vi "BRig_RT__Case_Exp__State_CuePre.vi"(0 "input_dataCurrent":u16[](array[numeric]), 1 "input_dataTrial":u16[][](array[numeric]), 6 "input_I_lick":bool, 7 "input_dataExp":u16[](array[numeric]), 9 "input_arrTrig":bool[](array[boolean])) -> (12 "output_state":T1, 13 "output_arrTrig":bool[](array[boolean]), 14 "output_dataCurrent":u16[](array[numeric]), 15 "output_dataTrial":u16[][](array[numeric]))   [LabVIEW 2014]
uses:
  myRIO_BRig_RT__Case_Exp_stateList.ctl
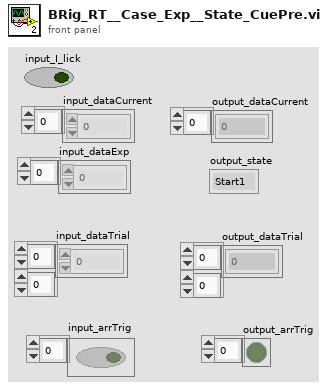
[diagram p1: front panel]
types:
  T1 = typedef "myRIO_BRig_RT__Case_Exp_stateList.ctl" = enum16{"Start1", "Start2", "Start3", "saveSettings1", "saveSettings2", "saveSettings3", "saveSettings4", "saveSettings_LC_ENL_l1", "saveSettings_LC_ENL_l2", "saveSettings_LC_Cue_l1", "saveSettings_LC_Cue_l2", "saveSettings6_LC_l1_Other", "SaveSettings6_LC_l2_Other", "setSettings_Audio", "setSettings_Laser", "initBlock_pre", "initBlock", "initBlock2", "initBlock_post", "initTrial_pre", "initTrial", "initTrial2", "initTrial3", "initTrial4", "initTrial_LC_ENL1", "initTrial_LC_Cue1", "initTrial_LC_Cue1_2", "initTrial_LC_Sel", "initTrial_post", "ENL1_pre", "ENL1", "ENL1_post", "ENL1Penalty_pre", "ENL1Penalty", "ENL2_pre", "ENL2", "ENL2Penalty_pre", "ENL2Penalty", "Cue1_pre", "Cue1", "Cue1_post", "Cue1Penalty_pre", "Cue1Penalty", "Cue2_pre", "Cue2", "Cue2Penalty_pre", "Cue2Penalty", "Selection_pre", "Selection", "Select_post", "SelectReward_pre", "SelectReward", "SelectRewardPost_pre", "SelectRewardPost", "SelectWrong_pre", "SelectWrong", "SelectWrong_post", "SelectTimeout_pre", "SelectTimeout", "SelectTimeout_post", "endTrial_pre", "endTrial1", "endTrial2", "endTrial3", "endTrial_post", "endBlock_pre", "endBlock", "endBlock_post", "endExp", "commConnect", "commUpload_pre", "commUpload_dataBlock", "commUpload_dataCurrent", "commUpload_dataExp", "commUpload_dataLC", "commUpload_dataTrial", "commUpload_post", "saveData_pre", "saveData_dataBlock", "saveData_dataCurrent", "saveData_dataExp", "saveData_dataLC", "saveData_dataTrial", "saveData_post", "empty_endBlock1", "empty_endBlock2", "empty_endTrial1", "empty_endTrial2", "empty_endTrial3", "empty_endTrial4", "empty_endTrial5", "dummyState", "dummyState_endBlock", "FreeReward_pre", "FreeReward", "FreeRewardPost_pre", "FreeRewardPost"}
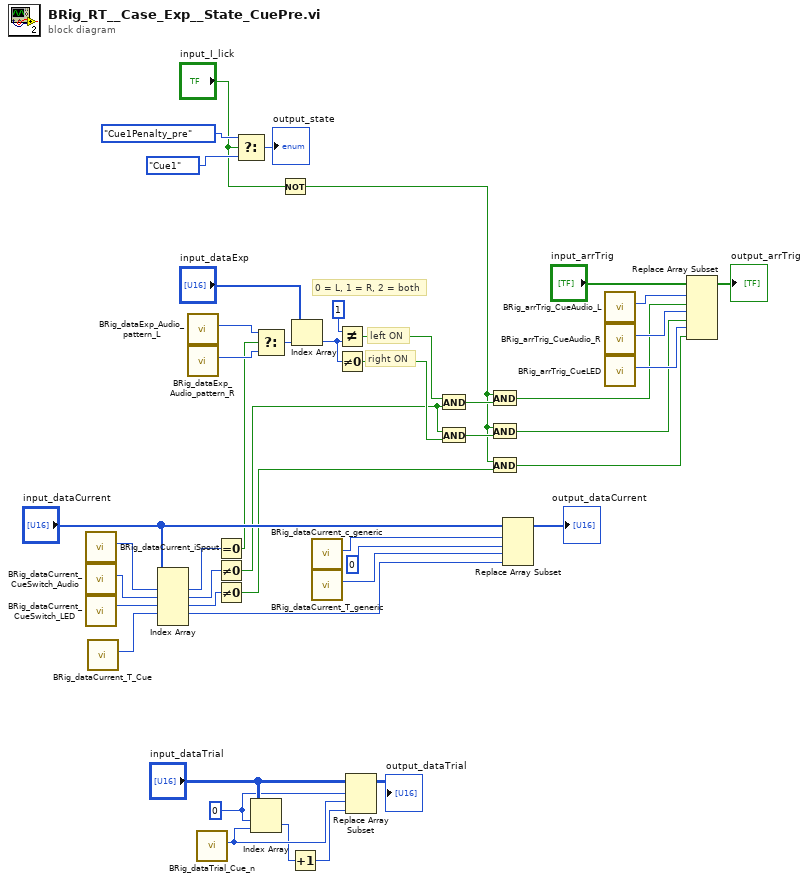
[diagram p0: block diagram]
diagram:
  w1 = 0
  # "right ON"
  # "left ON"
  # "0 = L, 1 = R, 2 = both"
  n1 = call "BRig_dataCurrent_iSpout.vi"() -> ("output_iSpout"=w24:i32)  [unwired: 11 in]
  n2 = call "BRig_dataCurrent_CueSwitch_Audio.vi"() -> ("output_CueSwitch_Audio"=w28:i32)  [unwired: 11 in]
  n3 = call "BRig_dataCurrent_CueSwitch_LED.vi"() -> ("output_CueSwitch_LED"=w29:i32)  [unwired: 11 in]
  n4 = call "BRig_dataCurrent_T_Cue.vi"() -> ("output_T_Cue"=w34:i32)  [unwired: 11 in]
  n5 = Index Array(array="input_dataCurrent", index #1=w24, index #2=w28, index #3=w29, index #4=w34) -> (element #1=w23:u16, element #2=w27:u16, element #3=w26:u16, element #4=w30:u16)  [unwired: 1 in, 1 out]
  n6 = call "BRig_dataExp_Audio_pattern_L.vi"() -> ("output_Audio_sp__L"=w39:i32)  [unwired: 11 in]
  n7 = call "BRig_dataExp_Audio_pattern_R.vi"() -> ("output_Audio_sp__R"=w40:i32)  [unwired: 11 in]
  n8 = call "BRig_dataTrial_Cue_n.vi"() -> ("output_Cue_n"=w13:i32)  [unwired: 11 in]
  n9 = Equal To 0?(x=w23) -> (x = 0?=w22:bool)
  n10 = Not Equal To 0?(x=w27) -> (x != 0?=w25:bool)
  n11 = Not Equal To 0?(x=w26) -> (x != 0?=w18:bool)
  n12 = Select(t=myRIO_BRig_RT__Case_Exp_stateList."Cue1Penalty_pre" ("Enum"), s="input_I_lick", f=myRIO_BRig_RT__Case_Exp_stateList."Cue1" ("Enum")) -> (s? t:f=→"output_state":T1)
  n13 = Index Array(array="input_dataTrial", index (row)=w1, index (col)=w13) -> (element=w12:u16)
  n14 = Select(t=w39, s=w22, f=w40) -> (s? t:f=w41:i32)
  n15 = Not(x="input_I_lick") -> (.not. x?=w17:bool)
  n16 = Increment(x=w12) -> (x+1=w11:u16)
  n17 = Index Array(array="input_dataExp", index=w41) -> (element=w15:u16)
  n18 = call "BRig_dataCurrent_c_generic.vi"() -> ("output_count_generic"=w33:i32)  [unwired: 11 in]
  n19 = call "BRig_dataCurrent_T_generic.vi"() -> ("output_T_generic"=w32:i32)  [unwired: 11 in]
  n20 = Not Equal?(x=u16 1 ("y"), y=w15) -> (x != y?=w37:bool)
  n21 = Not Equal To 0?(x=w15) -> (x != 0?=w36:bool)
  n22 = Replace Array Subset(array="input_dataTrial", new element=w11, index (row)=w1, index (col)=w13) -> (→"output_dataTrial":u16[][])
  n23 = And(x=w37, y=w25) -> (x .and. y?=w20:bool)
  n24 = And(x=w25, y=w36) -> (x .and. y?=w19:bool)
  n25 = And(x=w17, y=w20) -> (x .and. y?=w3:bool)
  n26 = And(x=w17, y=w19) -> (x .and. y?=w4:bool)
  n27 = And(x=w17, y=w18) -> (x .and. y?=w5:bool)
  n28 = Replace Array Subset(array="input_dataCurrent", new element #1=u16 0 ("new element/subarray"), index #1=w33, new element #2=w30, index #2=w32) -> (→"output_dataCurrent":u16[])
  n29 = call "BRig_arrTrig_CueAudio_L.vi"() -> ("output_CueAudio_L"=w8:i32)  [unwired: 11 in]
  n30 = call "BRig_arrTrig_CueAudio_R.vi"() -> ("output_CueAudio_R"=w7:i32)  [unwired: 11 in]
  n31 = call "BRig_arrTrig_CueLED.vi"() -> ("output_CueLED"=w6:i32)  [unwired: 11 in]
  n32 = Replace Array Subset(array="input_arrTrig", new element #1=w3, index #1=w8, new element #2=w4, index #2=w7, new element #3=w5, index #3=w6) -> (→"output_arrTrig":bool[])
